vi "Execute Msg.vi"(7 "Actor in":refnum<class "Actor.lvclass">, 8 "Error in":errorcluster, 11 "Stop Msg in":refnum<class "--Stop Msg.lvclass">) -> (0 "Error out":errorcluster, 2 "Msg Output":refnum<class "Msg Output.lvclass">, 5 "Actor out":refnum<class "Actor.lvclass">)   [LabVIEW 2025, in "jettl.lvlib" / "Stop jettl Msg.lvlib" / "--Stop Msg.lvclass"]
uses:
  --Stop Msg.lvclass
  Actor/Actor.lvclass
  Msg Output/Msg Output.lvclass
  Stop jettl Msg/Stop jettl Msg.lvclass
  --Stop Msg.lvclass/--Stop Msg.ctl
  --Stop Msg Output/--Stop Msg Output.lvclass
  C:/git/jettl/src/jettl/jettl/Msg Output/Msg Output.lvclass
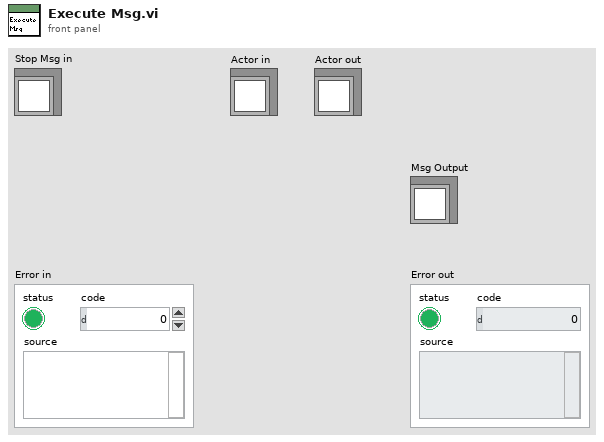
[diagram p1: front panel]
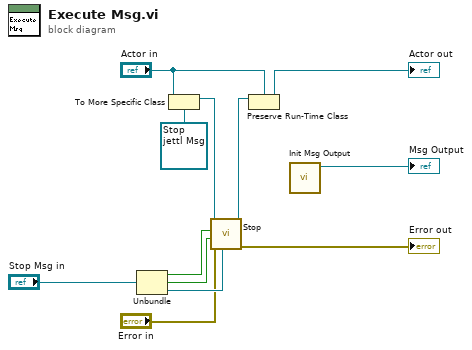
[diagram p0: block diagram]
diagram:
  n1 = Unbundle "Unbundle"("Stop Msg in") -> (w5:bool, w2:bool, w3:refnum<class "Teller.lvclass">)
  n2 = To More Specific Class(target class=refnum<class "Stop jettl Msg.lvclass"> refnum ("Destroy.lvlib:Destroy.lvclass"), reference="Actor in") -> (specific class reference=w8:refnum<class "Stop jettl Msg.lvclass">)  [unwired: 1 in, 1 out]
  n3 = call-dynamic "Stop.vi"("Teller"=w3, "Error in"="Error in", "Parent Stopped"=w2, "Safe Stop"=w5, "Stop jettl Msg in"=w8) -> ("Error out"=→"Error out":errorcluster, "Stop jettl Msg out"=w7:refnum<class "Stop jettl Msg.lvclass">)  [unwired: 5 in]
  n4 = Preserve Run-Time Class(object in=w7, 2:"Actor in") -> (object out=→"Actor out":refnum<class "Actor.lvclass">)  [unwired: 1 in, 1 out]
  n5 = call "Init Msg Output.vi"() -> ("Stop Msg Output out"=→"Msg Output":refnum<class "--Stop Msg Output.lvclass">)  [unwired: 11 in]
